vi "setSlitPosition.vi"(8 "error in (no error)":errorcluster, 10 "position":T1, 11 "Monochromator in":refnum<class "Monochromator.lvclass">) -> (0 "error out":errorcluster, 3 "Monochromator out":refnum<class "Monochromator.lvclass">)   [LabVIEW 2016, in "Monochromator.lvclass"]
uses:
  Monochromator.lvclass
  Typedefs/slit.ctl
  Typedefs/SlitType.ctl
  Typedefs/slitPosition.ctl
  Monochromator.lvclass/Monochromator.ctl
  Typedefs/AckType.ctl
  MonoStates/MonoState/MonoState.lvclass
  MonoCommunicator/MonoCommunicator.lvclass
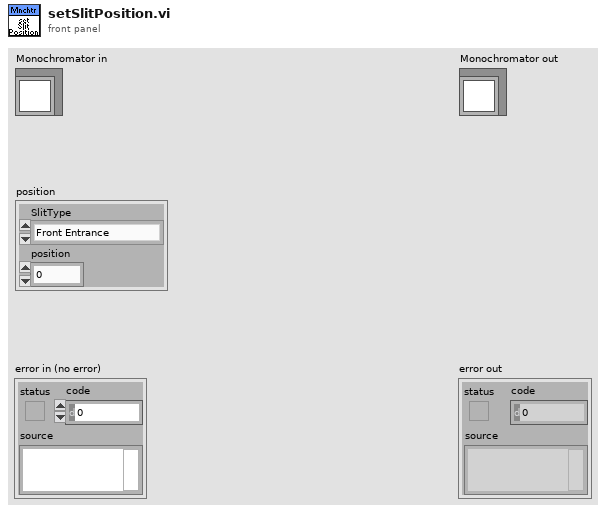
[diagram p1: front panel]
types:
  T1 = typedef "slit.ctl" = cluster{"SlitType":T2, "position":T3}
  T2 = typedef "SlitType.ctl" = enum16{"Front Entrance", "Side Entrance", "Front Exit", "Side Exit", "First Intermediate", "Second Intermediate"}
  T3 = typedef "slitPosition.ctl" = dbl
  T4 = typedef "AckType.ctl" = enum16{"OK", "OutOfRange", "Unknown", "Busy", "Rejected"}
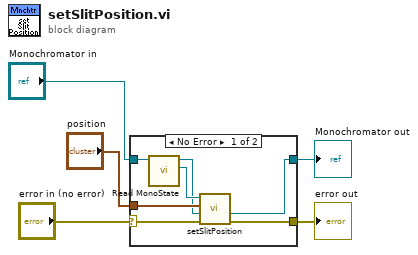
[diagram p0: block diagram]
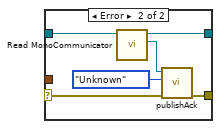
[diagram p2: hidden frame]
diagram:
  n1 = case shown="No Error" "error in (no error)" {
    selector: "error in (no error)" -> [w10 w16]
    tunnel: [w9 w13] -> w4
    tunnel: [w8 w14] -> w2
    tunnel: "Monochromator in" -> [w12 w15]
    tunnel: "position" -> [w11 _]
    frame No Error {
      n2 = call "Read MonoState.vi"("Monochromator in"=w12) -> ("MonoState.lvclass"=w7:refnum<class "MonoState.lvclass">, "Monochromator out"=w6:refnum<class "Monochromator.lvclass">)  [unwired: 8 in, 1 out]
      n3 = call-dynamic "setSlitPosition.vi"("error in (no error)"=w10, "Monochromator in"=w6, "position"=w11, "MonoState in"=w7) -> ("error out"=w9:errorcluster, "Monochromator out"=w8:refnum<class "Monochromator.lvclass">)  [unwired: 5 in, 1 out]
    }
    frame Error {
      n4 = call "Read MonoCommunicator.vi"("Monochromator in"=w15) -> ("MonoCommunicator.lvclass"=w17:refnum<class "MonoCommunicator.lvclass">, "Monochromator out"=w14:refnum<class "Monochromator.lvclass">)  [unwired: 8 in, 1 out]
      n5 = call "publishAck.vi"("error in (no error)"=w16, "AckType"=AckType."Unknown", "MonoCommunicator in"=w17) -> ("error out"=w13:errorcluster)  [unwired: 7 in, 1 out]
    }
  }
  "error out" <- w4
  "Monochromator out" <- w2
